vi "公式写入.vi"(7 "公式":cluster{"X^2":dbl, "X":dbl, "b":dbl}, 8 "error in (no error)":errorcluster caption="错误输入（无错误）", 9 "量程":enum16{"低量程", "高量程"}(ring), 10 "测量模式":T1(ring), 11 "测量参数":u16(ring) items=["总磷"=1, "总氮"=2, "氨氮"=3, "COD"=22]) -> (0 "error out":errorcluster caption="错误输出")   [LabVIEW 2016, in "斯坦道总磷.lvlib"]
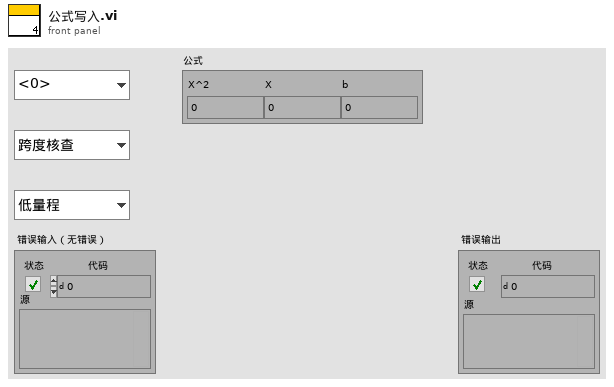
[diagram p1: front panel]
types:
  T1 = enum16{"跨度核查", "水样测量", "零点核查", "标样核查", "加标回收", "快捷测试", "空白校准", "标样校准"}
  T2 = typedef "SingleStepTestV3.lvlib/SingleStepTestV3.lvclass/仪器版本.ctl" = enum16{"V3.1版", "V4版", "V3版", "V4.2版"}
  T3 = cluster{"测量参数":u16, "测量模式":enum16{"跨度核查", "水样测量", "零点核查", "标样核查", "加标回收", "快捷测试", "空白校准", "标样校准"}, "量程":enum16{"低量程", "高量程"}}
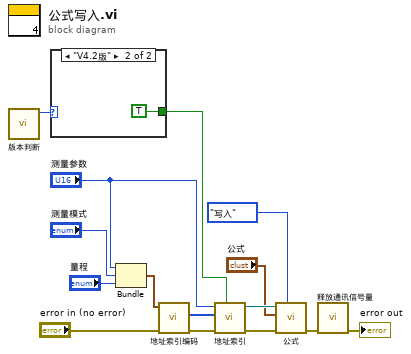
[diagram p0: block diagram]
diagram:
  n1 = call "版本判断.vi"() -> ("仪器版本"=w9:T2)  [unwired: 11 in]
  n2 = case shown="\"V4.2版\"" w9 {
    tunnel: [_ TRUE] -> w8
    frame "V3.1版", Default {
    }
    frame "V4.2版" {
    }
  }
  n3 = Bundle("测量参数"="测量参数", "测量模式"="测量模式", "量程"="量程") -> (w4:T3)  [unwired: 1 in]
  n4 = call "地址索引编码.vi"("error in (no error)"="error in (no error)", "参数簇"=w4) -> ("error out"=w1:errorcluster, "数组"=w3:u16[])  [unwired: 8 in]
  n5 = call "地址索引.vi"("4.2写公式？"=w8, "error in (no error)"=w1, "values"=w3, "测量参数"="测量参数") -> ("error out"=w14:errorcluster, "MB session out"=w15:refnum<class "MB_Master.lvclass">)  [unwired: 6 in]
  n6 = call "公式.vi"("功能"=enum16{"读取", "写入"}."写入", "error in (no error)"=w14, "公式写入"="公式", "MB session in"=w15) -> ("error out"=w12:errorcluster)  [unwired: 5 in, 2 out]
  n7 = call "释放通讯信号量.vi"("error in (no error)"=w12) -> ("error out"=→"error out":errorcluster)  [unwired: 10 in]
